vi "人脸区域去背景_example.vi"() -> ()   [LabVIEW 2017]
doc: "This example illustrates Grab cut algorithm in OpenCV. Use this example to understand passing NI Vision images and LabVIEW cluster to OpenCV wrapper dll."
uses:
  <vilib>/vision/NI_Vision_Development_Module.lvlib
panel:
  out "Rectangle":T1 {"Rotation" min=-90.0 max=90.0 step=1.0 format="%.2f"; "Left" scale=0.0..1024.0; "Right" scale=0.0..1024.0}
  out "Segmented Image":T2(plugin-control)
  out "Source Image":T2(plugin-control)
  # "Overview: Demonstrates how to use OpenCV Grabcut algorithm \nRequirements: Vision Development Module\nInstructions:\n1. Draw ROI on object in Source Image for segmentation\n2. Run the VI"
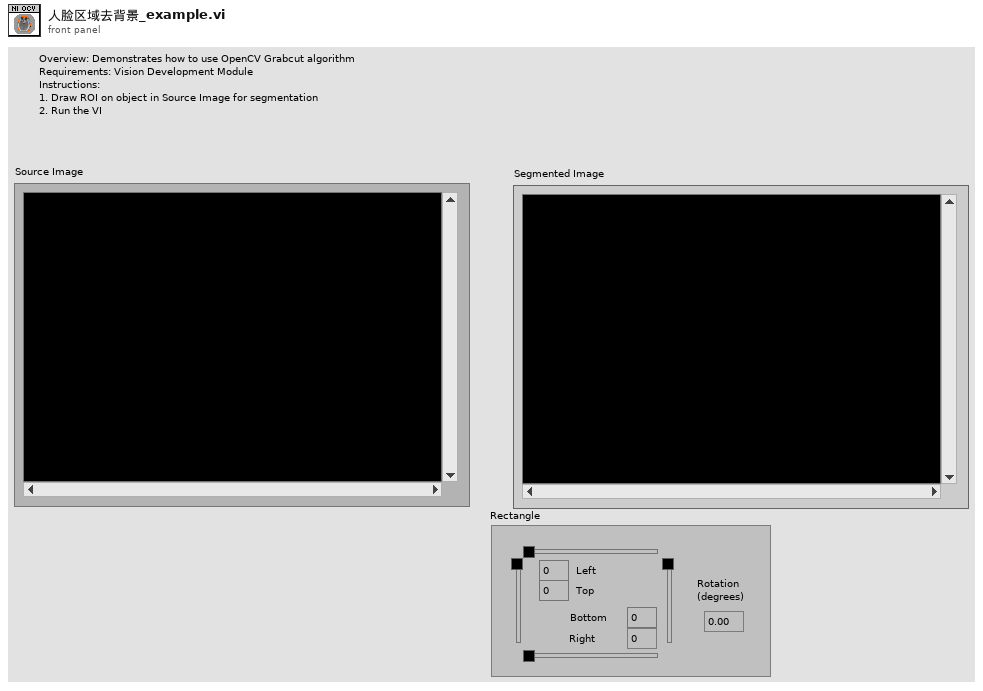
[diagram p1: front panel]
types:
  T1 = typedef "IMAQ Rectangle" = cluster{"Left":i32, "Top":i32, "Right":i32, "Bottom":i32, "Rotation":dbl}
  T2 = typedef "IMAQ Image.ctl" = refnum<image>
  T3 = enum32{"Average", "Min", "Max", "Clear  if < ", "Clear  if < or =", "Clear  if =", "Clear  if > or =", "Clear  if >"}
  T4 = typedef "Image Type" = u32
  T5 = cluster{"Global Rectangle":i32[], "Contours":cluster{"Contour Type":u32, "ROI Type":u32, "Points":i32[]}[]}
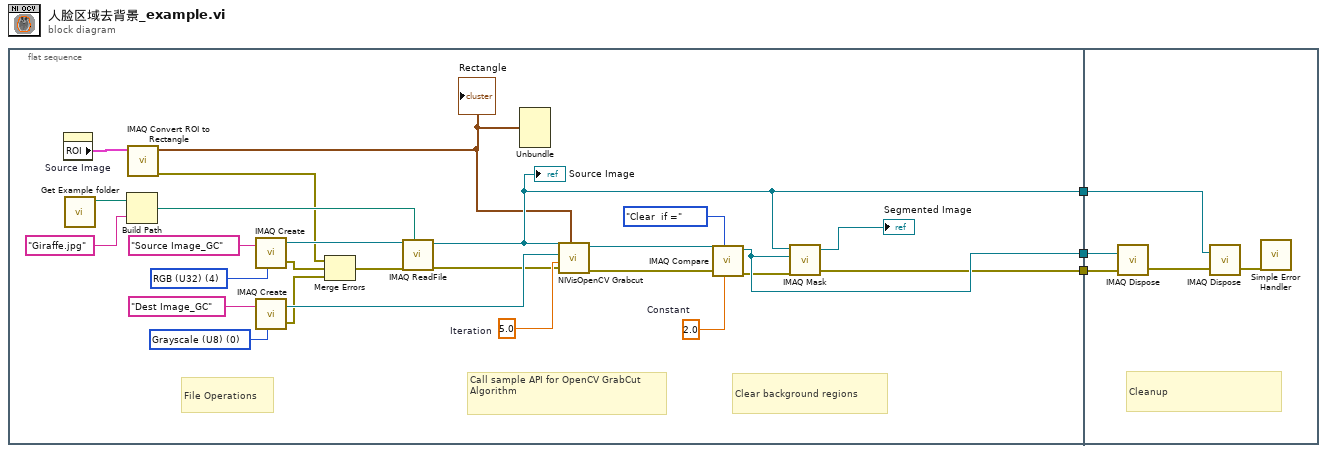
[diagram p0: block diagram]
diagram:
  n1 = flat-sequence {
    tunnel: [w18] -> w3
    tunnel: [w16] -> w2
    tunnel: [w14] -> w1
    tunnel: w3 -> [w30]
    tunnel: w2 -> [w31]
    tunnel: w1 -> [w32]
    frame #0 {
      w19 = sgl 2.0  # Constant
      w22 = 5.0  # Iteration
      w25 = T4 0 items=["Grayscale (U8)", "Grayscale (I16)", "Grayscale (SGL)", "Complex (CSG)", "RGB (U32)", "HSL (U32)", "RGB (U64)", "Grayscale (U16)"] ("Image Type")
      w28 = T4 4 items=["Grayscale (U8)", "Grayscale (I16)", "Grayscale (SGL)", "Complex (CSG)", "RGB (U32)", "HSL (U32)", "RGB (U64)", "Grayscale (U16)"] ("Image Type")
      # "Clear background regions"
      # "Call sample API for OpenCV GrabCut Algorithm"
      # "File Operations"
      n2 = property on="Source Image" class="ImageControl"() -> ("ROI"=w8:T5)  [unwired: 2 in, 2 out]
      n3 = call "Get Example folder.vi"() -> ("Example Image Path"=w13:path)  [unwired: 11 in]
      n4 = Build Path(base path=w13, name or relative path="Giraffe.jpg" ("Image Name")) -> (appended path=w11:path)
      n5 = call "IMAQ Convert ROI to Rectangle"("ROI Descriptor"=w8) -> ("error out"=w5:errorcluster, "Rectangle"=w4:T1)  [unwired: 8 in]
      "Rectangle" <- w4
      n6 = call "IMAQ Create"("Image Name"="Source Image_GC", "Image Type"=w28) -> ("New Image"=w29:T2, "error out"=w6:errorcluster)  [unwired: 3 in]
      n7 = call "IMAQ Create"("Image Name"="Dest Image_GC", "Image Type"=w25) -> ("New Image"=w23:T2, "error out"=w7:errorcluster)  [unwired: 3 in]
      n8 = Merge Errors(w5, w6, w7) -> (w24:errorcluster)
      n9 = call "IMAQ ReadFile"("File Path"=w11, "error in (no error)"=w24, "Image"=w29) -> ("error out"=w9:errorcluster, "Image Out"=w18:T2)  [unwired: 4 in, 3 out]
      "Source Image" <- w18
      n10 = Unbundle(w4) -> ()  [unwired: 5 out]
      n11 = call <vilib>:"NIVisOpenCV Grabcut.vi"("Rectangle"=w4, "error in (no error)"=w9, "Iteration"=w22, "Image Foreground Mask"=w23, "Image Src"=w18) -> ("error out"=w10:errorcluster, "Image Foreground Mask Out"=w21:T2)  [unwired: 5 in]
      n12 = call "IMAQ Compare"("Constant"=w19, "Operator"=T3."Clear  if =", "error in (no error)"=w10, "Image Src A"=w21) -> ("error out"=w15:errorcluster, "Image Dst Out"=w16:T2)  [unwired: 6 in]
      n13 = call "IMAQ Mask"("error in (no error)"=w15, "Image Mask"=w16, "Image Src"=w18) -> ("error out"=w14:errorcluster, "Image Dst Out"=→"Segmented Image":T2)  [unwired: 2 in]
    }
    frame #1 {
      # "Cleanup"
      n14 = call "IMAQ Dispose"("Image"=w31, "error in (no error)"=w32) -> ("error out"=w33:errorcluster)  [unwired: 4 in]
      n15 = call "IMAQ Dispose"("Image"=w30, "error in (no error)"=w33) -> ("error out"=w34:errorcluster)  [unwired: 4 in]
      n16 = call <vilib>:"Simple Error Handler.vi"("error in (no error)"=w34) -> ()  [unwired: 4 in, 5 out]
    }
  }
